vi "Transform.vi"(10 "SampleRate":dbl, 11 "TimeDomainIn":cdb[](array[numeric])) -> (1 "Complex":cdb[](array[numeric]), 2 "df (Hz)":dbl, 3 "AmplitudeSpectrum":dbl[](array[numeric]), 4 "TheEugeneHong":dbl[][](array[numeric]), 5 "Quadrature":dbl[](array[numeric]), 7 "InPhase":dbl[](array[numeric]))   [LabVIEW 2018]
doc: "Apply window\nFFT\nCalculate Vrms^2 spectrum"
uses:
  <vilib>/Analysis/4window.llb/Hanning Window (CDB).vi
  <vilib>/Analysis/2dsp.llb/Complex FFT.vi
  <vilib>/Analysis/4window.llb/AllCosWindow (CDB).vi
  <vilib>/Analysis/NI_AALPro.lvlib
panel:
  out "error":i32
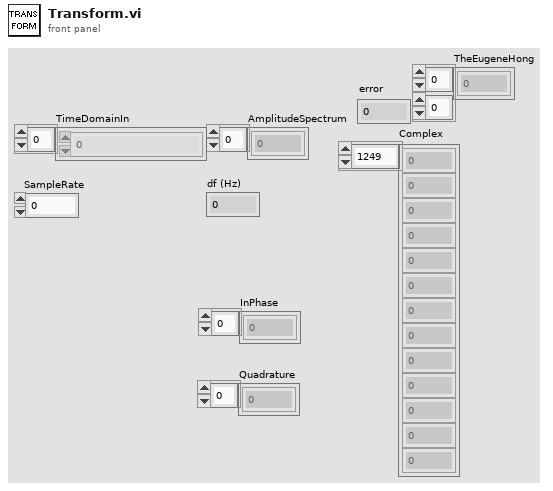
[diagram p1: front panel]
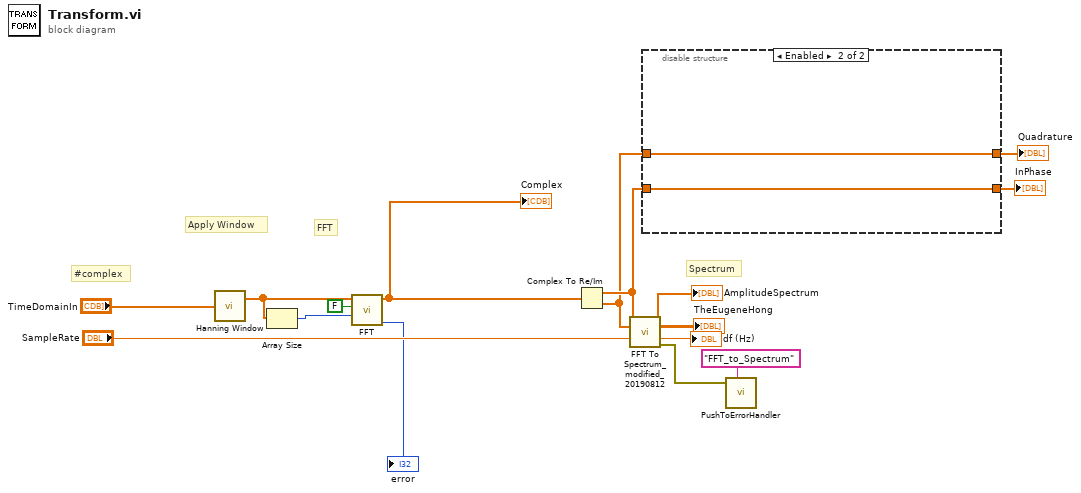
[diagram p0: block diagram]
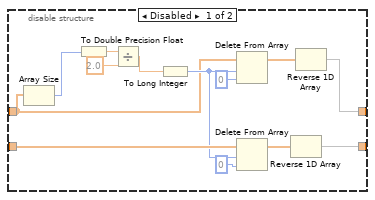
[diagram p2: hidden frame]
diagram:
  # "#complex"
  # "Spectrum"
  # "FFT"
  # "Apply Window"
  n1 = call-poly <vilib>:"Hanning Window.vi"("X"="TimeDomainIn") -> ("Windowed X"=w4:cdb[])  [unwired: 1 out]
  n2 = Array Size(array=w4) -> (size(s)=w5:i32)
  n3 = call-poly <vilib>:"FFT.vi"("FFT size"=w5, "shift?"=FALSE, "X"=w4) -> ("error"=→"error":i32, "FFT {X}"=w6:cdb[])  [unwired: 7 in]
  "Complex" <- w6
  n4 = Complex To Re/Im(x + iy=w6) -> (x=w10:dbl[], y=w7:dbl[])
  n5 = call "FFT To Spectrum_modified_20190812.vi"("real FFT data"=w10, "imaginary FFT data"=w7, "sample rate (S/s)"="SampleRate") -> ("spectrum out (V)"=→"AmplitudeSpectrum":dbl[], "TheEugeneHong"=→"TheEugeneHong":dbl[][], "df (Hz)"=→"df (Hz)":dbl, "error out"=w2:errorcluster)  [unwired: 9 in]
  n6 = disable-structure shown="Enabled" {
    disable-tunnel: w10 -> [w24 w30]
    disable-tunnel: [w19 w31] -> w9
    disable-tunnel: [w18 w30] -> w8
    disable-tunnel: w7 -> [w17 w31]
    frame Disabled {
      n7 = Array Size(array=w17) -> (size(s)=w29:i32)
      n8 = To Double Precision Float(number=w29) -> (double precision float=w28:dbl)
      n9 = Divide(x=w28, y=2.0) -> (x/y=w26:dbl)
      n10 = To Long Integer(number=w26) -> (32bit integer=w20:i32)
      n11 = Delete From Array(array=w17, length=w20, index=0) -> (array with subset deleted=w25:dbl[])  [unwired: 1 out]
      n12 = Delete From Array(array=w24, length=w20, index=0) -> (array with subset deleted=w23:dbl[])  [unwired: 1 out]
      n13 = Reverse 1D Array(array=w23) -> (reversed array=w18:dbl[])
      n14 = Reverse 1D Array(array=w25) -> (reversed array=w19:dbl[])
    }
    frame Enabled {
    }
  }
  "InPhase" <- w8
  "Quadrature" <- w9
  n15 = call "PushToErrorHandler.vi"("ErrorIn"=w2, "ErrorLocation"="FFT_to_Spectrum") -> ()  [unwired: 5 in, 1 out]
